vi "GObjectFactory_BD.vi"(8 "error in":errorcluster, 11 "reference":refnum<vi>) -> (0 "error out":errorcluster, 3 "GObject out":refnum<class "GObject.lvclass">)   [LabVIEW 2014, in "Raspberry Pi Compatible Compiler for LabVIEW.lvlib" / "GObject.lvclass"]
uses:
  GObject.lvclass
  Wire/Wire.lvclass
  Node/Node.lvclass
  Terminal/Terminal.lvclass
  Constant/Constant.lvclass
  Diagram/Diagram.lvclass
  Tunnel/Tunnel.lvclass
  FlatSequence/FlatSequence.lvclass
  FlatSequenceInnerTunnel/FlatSequenceInnerTunnel.lvclass
  FlatSequenceOuterTunnel/FlatSequenceOuterTunnel.lvclass
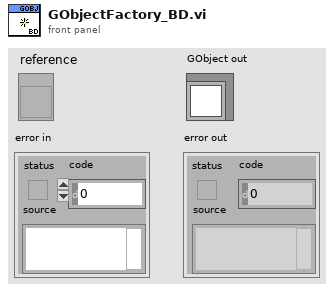
[diagram p1: front panel]
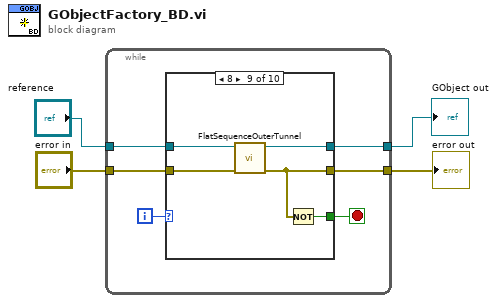
[diagram p0: block diagram]
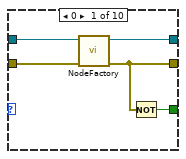
[diagram p2: hidden frame]
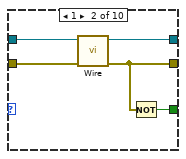
[diagram p3: hidden frame]
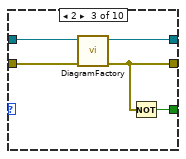
[diagram p4: hidden frame]
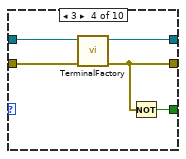
[diagram p5: hidden frame]
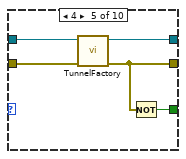
[diagram p6: hidden frame]
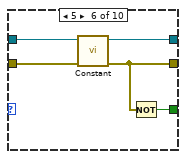
[diagram p7: hidden frame]
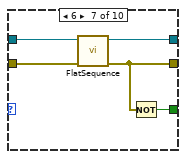
[diagram p8: hidden frame]
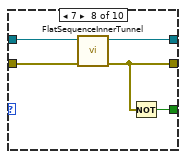
[diagram p9: hidden frame]
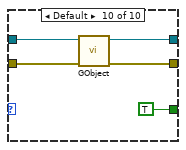
[diagram p10: hidden frame]
diagram:
  n1 = while {
    tunnel: "reference" -> [w9]
    tunnel: "error in" -> [w8]
    tunnel: [w7] -> w1
    tunnel: [w6] -> w2
    i -> [w10]
    stop <- w5 stop-if-true
    n2 = case shown="8" w10 {
      tunnel: w9 -> [w14 w19 w24 w29 w34 w39 w44 w49 w54 w58]
      tunnel: w8 -> [w15 w20 w25 w30 w35 w40 w45 w50 w55 w59]
      tunnel: [w11 w16 w21 w26 w31 w36 w41 w46 w51 w57] -> w7
      tunnel: [w13 w18 w23 w28 w33 w38 w43 w48 w53 w60] -> w6
      tunnel: [w12 w17 w22 w27 w32 w37 w42 w47 w52 TRUE] -> w5
      frame 0 {
        n3 = call "NodeFactory.vi"("error in"=w15, "reference"=w14) -> ("error out"=w11:errorcluster, "Node out"=w13:refnum<class "Node.lvclass">)  [unwired: 8 in]
        n4 = Not(x=w11) -> (.not. x?=w12:bool)
      }
      frame 1 {
        n5 = call "Wire.vi"("error in"=w20, "reference"=w19) -> ("error out"=w16:errorcluster, "wire"=w18:refnum<class "Wire.lvclass">)  [unwired: 8 in]
        n6 = Not(x=w16) -> (.not. x?=w17:bool)
      }
      frame 2 {
        n7 = call "DiagramFactory.vi"("error in"=w25, "reference"=w24) -> ("error out"=w21:errorcluster, "Diagram out"=w23:refnum<class "Diagram.lvclass">)  [unwired: 8 in]
        n8 = Not(x=w21) -> (.not. x?=w22:bool)
      }
      frame 3 {
        n9 = call "TerminalFactory.vi"("error in"=w30, "reference"=w29) -> ("error out"=w26:errorcluster, "terminal"=w28:refnum<class "Terminal.lvclass">)  [unwired: 8 in]
        n10 = Not(x=w26) -> (.not. x?=w27:bool)
      }
      frame 4 {
        n11 = call "TunnelFactory.vi"("error in"=w35, "reference"=w34) -> ("error out"=w31:errorcluster, "Tunnel out"=w33:refnum<class "Tunnel.lvclass">)  [unwired: 8 in]
        n12 = Not(x=w31) -> (.not. x?=w32:bool)
      }
      frame 5 {
        n13 = call "Constant.vi"("error in"=w40, "reference"=w39) -> ("error out"=w36:errorcluster, "constant out"=w38:refnum<class "Constant.lvclass">)  [unwired: 8 in]
        n14 = Not(x=w36) -> (.not. x?=w37:bool)
      }
      frame 6 {
        n15 = call "FlatSequence.vi"("error in"=w45, "reference"=w44) -> ("error out"=w41:errorcluster, "Flat Sequence out"=w43:refnum<class "FlatSequence.lvclass">)  [unwired: 8 in]
        n16 = Not(x=w41) -> (.not. x?=w42:bool)
      }
      frame 7 {
        n17 = call "FlatSequenceInnerTunnel.vi"("error in"=w50, "reference"=w49) -> ("error out"=w46:errorcluster, "Tunnel out"=w48:refnum<class "FlatSequenceInnerTunnel.lvclass">)  [unwired: 8 in]
        n18 = Not(x=w46) -> (.not. x?=w47:bool)
      }
      frame 8 {
        n19 = call "FlatSequenceOuterTunnel.vi"("error in"=w55, "reference"=w54) -> ("error out"=w51:errorcluster, "Tunnel out"=w53:refnum<class "FlatSequenceOuterTunnel.lvclass">)  [unwired: 8 in]
        n20 = Not(x=w51) -> (.not. x?=w52:bool)
      }
      frame Default {
        n21 = call "GObject.vi"("error in"=w59, "reference"=w58) -> ("error out"=w57:errorcluster, "GObject out"=w60:refnum<class "GObject.lvclass">)  [unwired: 8 in]
      }
    }
  }
  "error out" <- w1
  "GObject out" <- w2
